vi "ImageCode.vi"() -> ()   [LabVIEW 2011]
uses:
  <vilib>/Rock Robotics/WPI/Camera/WPI_CameraImageSize.ctl
panel:
  out "Image Error Message":string="Timeout in Camera Communications"
  in  "Viewer":enum32{"Camera Image"}(tab)
  in  "Video Enable":bool=TRUE
  out "Camera Image":T1(plugin-control)
  out "Output String":string
  out "Length":i32
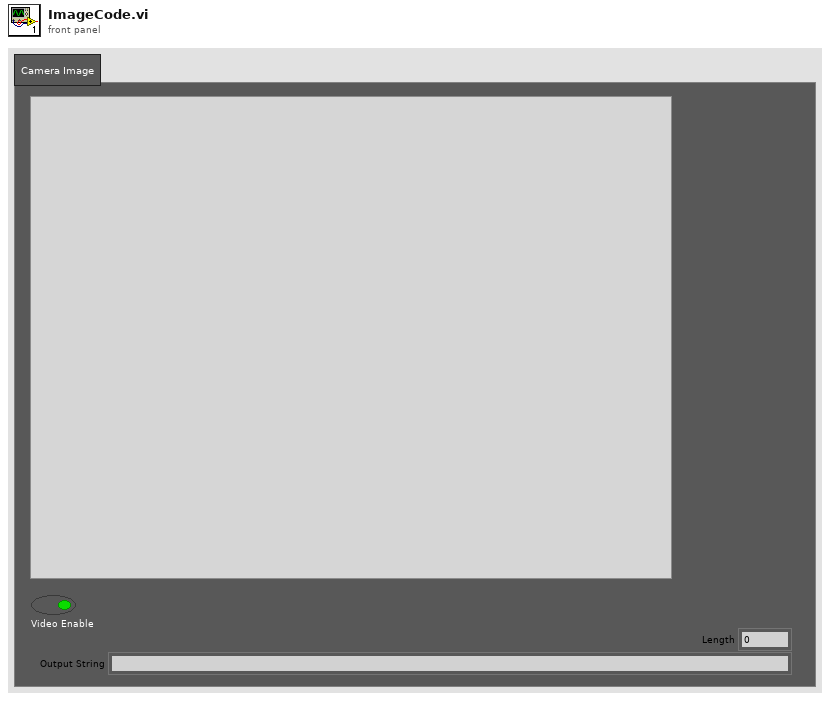
[diagram p1: front panel]
types:
  T1 = typedef "IMAQ Image.ctl" = refnum<image>
  T2 = typedef "Image Type" = u32
  T3 = cluster{"Left":i32, "Top":i32, "Right":i32, "Bottom":i32}
  T4 = typedef "WPI_CameraImageSize.ctl" = enum16{"640x480", "320x240", "160x120"}
  T5 = cluster{"fps":i32, "compression":i32, "Image Size":T4}
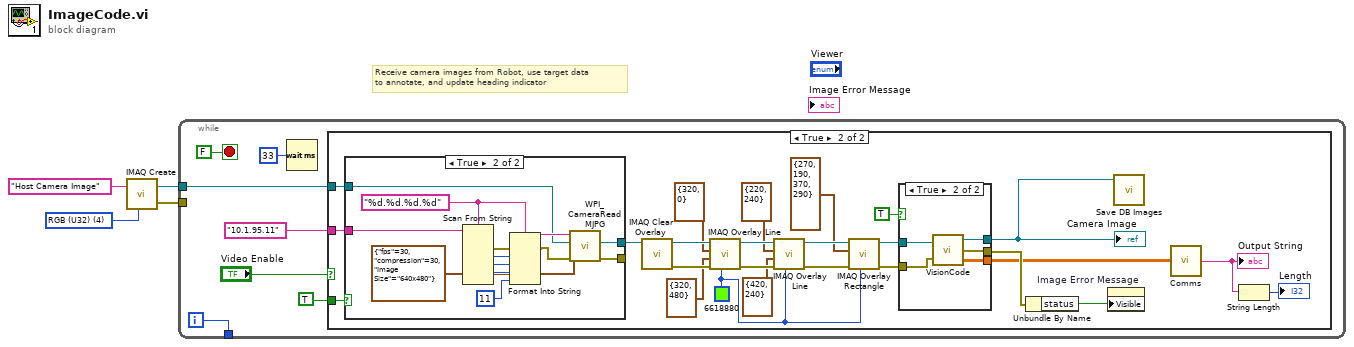
[diagram p0: block diagram]
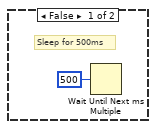
[diagram p2: hidden frame]
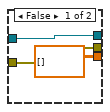
[diagram p3: hidden frame]
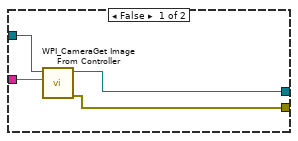
[diagram p4: hidden frame]
diagram:
  w4 = T2 4 items=["Grayscale (U8)", "Grayscale (I16)", "Grayscale (SGL)", "Complex (CSG)", "RGB (U32)", "HSL (U32)", "RGB (U64)"] ("Image Type")
  # "Receive camera images from Robot, use target data\nto annotate, and update heading indicator"
  n1 = call "IMAQ Create"("Image Name"="Host Camera Image", "Image Type"=w4) -> ("New Image"=w2:T1, "error out"=w1:errorcluster)  [unwired: 2 in, 1 out]
  n2 = while {
    tunnel: w2 -> [w9]
    tunnel: w1 -> [_]
    tunnel: [w6] -> _
    i -> [w6]
    stop <- FALSE stop-if-true
    n3 = Wait (ms)(milliseconds to wait=u32 33) -> ()  [unwired: 1 out]
    n4 = case shown="True" "Video Enable" {
      tunnel: "10.1.95.11" ("Robot IP Address") -> [_ w37]
      tunnel: w9 -> [_ w36]
      tunnel: TRUE -> [_ w33]
      frame False {
        # "Sleep for 500ms"
        n5 = Wait Until Next ms Multiple(millisecond multiple=u32 500) -> ()  [unwired: 1 out]
      }
      frame True {
        w16 = u32 6618880 ("Color")
        n6 = case shown="True" w33 {
          tunnel: w36 -> [w48 w56]
          tunnel: [w46 w54] -> _
          tunnel: [w47 w55] -> w34
          tunnel: w37 -> [w49 w59]
          frame False {
            n7 = call <vilib>:"WPI_CameraGet Image From Controller.vi"("Controller Address"=w49, "Image"=w48) -> ("error out"=w46:errorcluster, "Image Out"=w47:T1)  [unwired: 2 in, 6 out]
          }
          frame True {
            w51 = "%d.%d.%d.%d" ("format string")
            n8 = Scan From String(format string=w51, input string=w59) -> (error out=w58:errorcluster, output 1=w60:i32, output 2=w61:i32, output 3=w62:i32)  [unwired: 2 in, 7 out]
            n9 = Format Into String(format string=w51, error in=w58, w60, w61, w62, 11 ("IP Suffix:")) -> (resulting string=w57:string, error out=w53:errorcluster)  [unwired: 1 in]
            n10 = call <vilib>:"WPI_CameraRead MJPG.vi"("error in"=w53, "Camera Settings"=T5 {"fps"=30, "compression"=30, "Image Size"=enum."640x480"}, "Image"=w56, "address"=w57) -> ("error out"=w54:errorcluster, "Image Out"=w55:T1)  [unwired: 6 in]
          }
        }
        n11 = call "IMAQ Clear Overlay"("Image"=w34) -> ("error out"=w31:errorcluster, "Image Out"=w32:T1)  [unwired: 2 in, 7 out]
        n12 = call "IMAQ Overlay Line"("Color"=w16, "error in (no error)"=w31, "End Point"=cluster{"X":i32, "Y":i32} {"X"=320, "Y"=480}, "Start Point"=cluster{"X":i32, "Y":i32} {"X"=320, "Y"=0}, "Image"=w32) -> ("error out"=w27:errorcluster, "Image Out"=w28:T1)  [unwired: 5 in]
        n13 = call "IMAQ Overlay Line"("Color"=w16, "error in (no error)"=w27, "End Point"=cluster{"X":i32, "Y":i32} {"X"=420, "Y"=240}, "Start Point"=cluster{"X":i32, "Y":i32} {"X"=220, "Y"=240}, "Image"=w28) -> ("error out"=w23:errorcluster, "Image Out"=w24:T1)  [unwired: 5 in]
        n14 = call "IMAQ Overlay Rectangle"("Color"=w16, "error in (no error)"=w23, "Rectangle"=T3 {"Left"=270, "Top"=190, "Right"=370, "Bottom"=290}, "Image"=w24) -> ("error out"=w21:errorcluster, "Image Out"=w19:T1)  [unwired: 6 in]
        n15 = case shown="True" TRUE {
          tunnel: w21 -> [w39 w45]
          tunnel: [w39 w42] -> w20
          tunnel: w19 -> [w40 w44]
          tunnel: [w40 w43] -> w18
          tunnel: [dbl[][] [] ("Particle Measurements (Pixels)") w41] -> w15
          frame False {
          }
          frame True {
            n16 = call "VisionCode.vi"("Image Src"=w44, "error in (no error)"=w45) -> ("Image Out"=w43:T1, "error out"=w42:errorcluster, "Particle Measurements (Pixels)"=w41:dbl[][])
          }
        }
        "Camera Image" <- w18
        n17 = Unbundle By Name(w20) -> ("status"=w35:bool)
        n18 = property on="Image Error Message" class="Str"("Visible"=w35) -> ()  [unwired: 2 in, 2 out]
        n19 = call "Save DB Images.vi"("Image"=w18) -> ()  [unwired: 2 in, 1 out]
        n20 = call "Comms.vi"("Array"=w15) -> ("String"=w14:string)
        "Output String" <- w14
        n21 = String Length(string=w14) -> (length=→"Length":i32)
      }
    }
  }
